vi "Generate PPM Waveform.vi"(8 "error in (no error)":errorcluster, 9 "frequency (Hz)":dbl=50.0, 10 "Scale Factor":dbl=1.0, 11 "duty cycle (%)":dbl=12.5 min=2.5 max=25.0 format="%0.2f") -> (0 "error out":errorcluster, 1 "Waveform Graph":waveform(dbl)(graph), 2 "signal out":waveform(dbl), 3 "digital waveform":digitalwaveform(waveform)={"t0"=timestamp(0 s since 1904-01-01), "dt"=0.0, "Y"={"transitions"=[], "data"=[]}, "error"={"status"=FALSE, "code"=37421928, "source"=""}}, 4 "GraphMaxY":dbl)   [LabVIEW 2021]
uses:
  <vilib>/Waveform/DWDTOps.llb/DWDT Analog to Digital.vi
  <vilib>/measure/NI_MABase.lvlib
panel:
  # "50Hz for PPM\nControl for Testing"
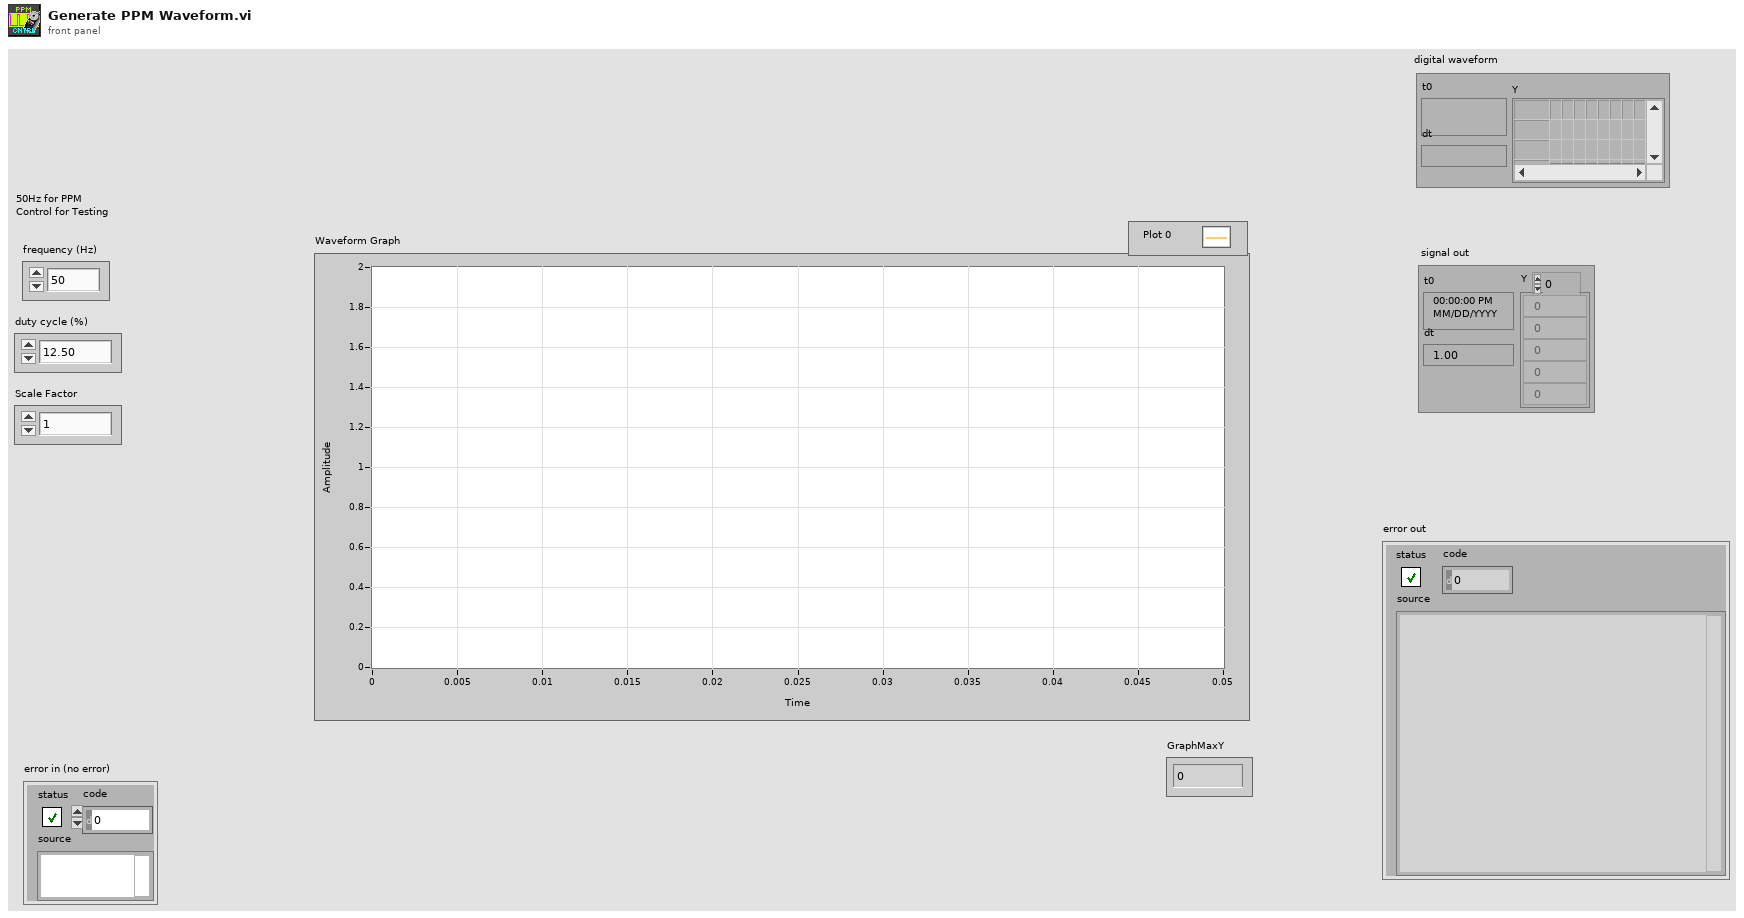
[diagram p1: front panel]
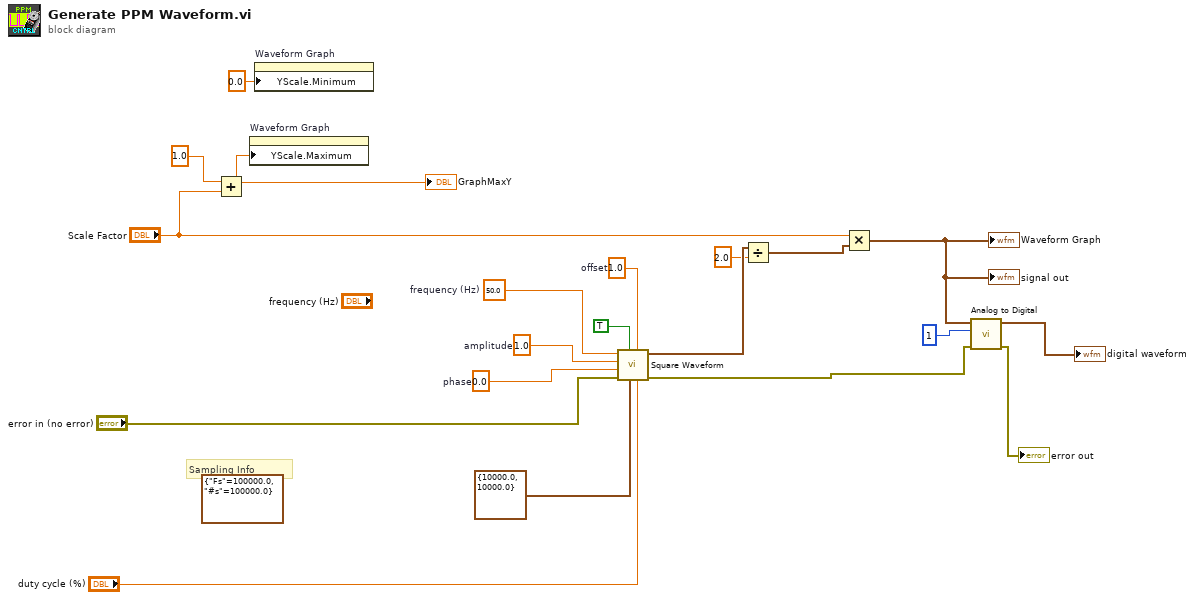
[diagram p0: block diagram]
diagram:
  (unwired) cluster{"Fs":dbl, "#s":dbl} {"Fs"=100000.0, "#s"=100000.0}
  w15 = 1.0  # offset
  w18 = 0.0  # phase
  w19 = 1.0  # amplitude
  w20 = 50.0  # frequency (Hz)
  # "Sampling Info"
  n1 = Add(x=1.0, y="Scale Factor") -> (x+y=w9:dbl)
  "GraphMaxY" <- w9
  n2 = property on="Waveform Graph" class="WFGraph (strict)"("YScale.Maximum"=w9) -> ()  [unwired: 2 in, 2 out]
  n3 = property on="Waveform Graph" class="WFGraph (strict)"("YScale.Minimum"=0.0 ("Y Scale.Range:Minimum")) -> ()  [unwired: 2 in, 2 out]
  n4 = call <vilib>:"Square Waveform.vi"("duty cycle (%)"="duty cycle (%)", "offset"=w15, "sampling info"=cluster{"Fs":dbl, "#s":dbl} {"Fs"=10000.0, "#s"=10000.0}, "reset signal"=TRUE, "error in (no error)"="error in (no error)", "phase"=w18, "amplitude"=w19, "frequency"=w20) -> ("error out"=w4:errorcluster, "signal out"=w13:waveform(dbl))  [unwired: 2 in]
  n5 = Divide(x=w13, y=2.0) -> (x/y=w11:waveform(dbl))
  n6 = Multiply(x="Scale Factor", y=w11) -> (x*y=w6:waveform(dbl))
  "signal out" <- w6
  "Waveform Graph" <- w6
  n7 = call-poly <vilib>:"Analog to Digital.vi"("error in (no error)"=w4, "resolution (16 bit)"=1, "analog waveform"=w6) -> ("error out"=→"error out":errorcluster, "digital waveform"=→"digital waveform":digitalwaveform)  [unwired: 5 in, 2 out]
